vi "Get 1553 Configuration.vi"() -> (3 "1553 Configuration":T1)   [LabVIEW 2020, in "AIM MIL-STD-1553 Engine.lvlib" / "Custom Device.lvlib"]
uses:
  Custom Device.lvlib
  1553 Configuration.ctl
  Major Frame Configuration.ctl
  Minor Frame Configuration.ctl
  Message Configuration.ctl
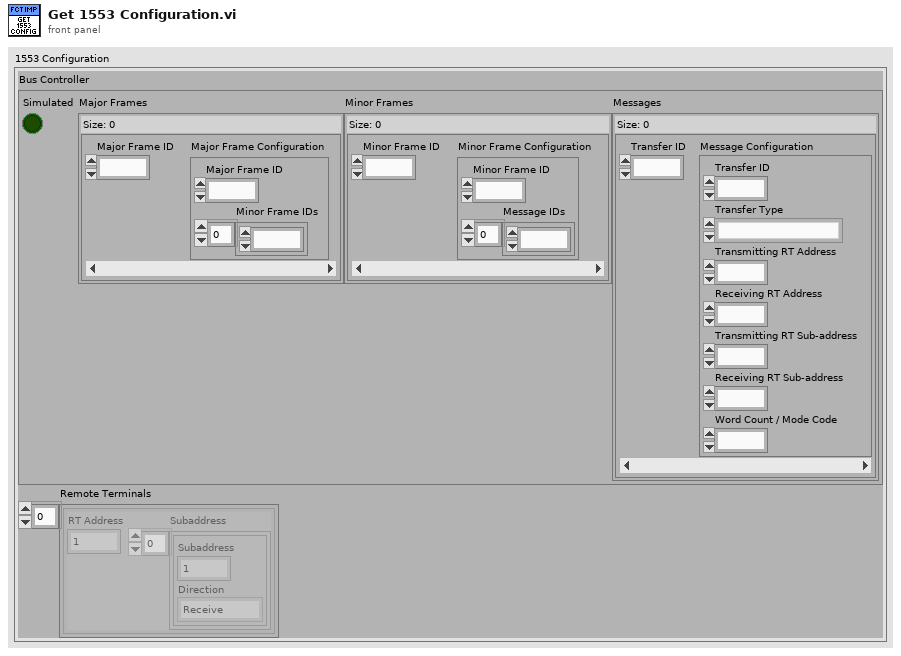
[diagram p1: front panel]
types:
  T1 = typedef "AIM MIL-STD-1553 Engine.lvlib/Custom Device.lvlib/1553 Configuration.ctl" = cluster{"Bus Controller":cluster{"Simulated":bool, "Major Frames":map{u16, T2}, "Minor Frames":map{u16, T3}, "Messages":map{u16, T4}}, "Remote Terminals":cluster{"RT Address":u8, "Subaddress":cluster{"Subaddress":u8, "Direction":enum16{"Receive", "Transmit"}}[]}[]}
  T2 = typedef "AIM MIL-STD-1553 Engine.lvlib/Custom Device.lvlib/Major Frame Configuration.ctl" = cluster{"Major Frame ID":u16, "Minor Frame IDs":u16[]}
  T3 = typedef "AIM MIL-STD-1553 Engine.lvlib/Custom Device.lvlib/Minor Frame Configuration.ctl" = cluster{"Minor Frame ID":u16, "Message IDs":u16[]}
  T4 = typedef "AIM MIL-STD-1553 Engine.lvlib/Custom Device.lvlib/Message Configuration.ctl" = cluster{"Transfer ID":u16, "Transfer Type":enum16{"BC to RT transfer", "RT to BC transfer", "RT to RT transfer"}, "Transmitting RT Address":u8, "Receiving RT Address":u8, "Transmitting RT Sub-address":u8, "Receiving RT Sub-address":u8, "Word Count / Mode Code":u8}
  T5 = cluster{"RT Address":u8, "Subaddress":cluster{"Subaddress":u8, "Direction":enum16{"Receive", "Transmit"}}[]}[]
  T6 = cluster{"Simulated":bool, "Major Frames":map{u16, T2}, "Minor Frames":map{u16, T3}, "Messages":map{u16, T4}}
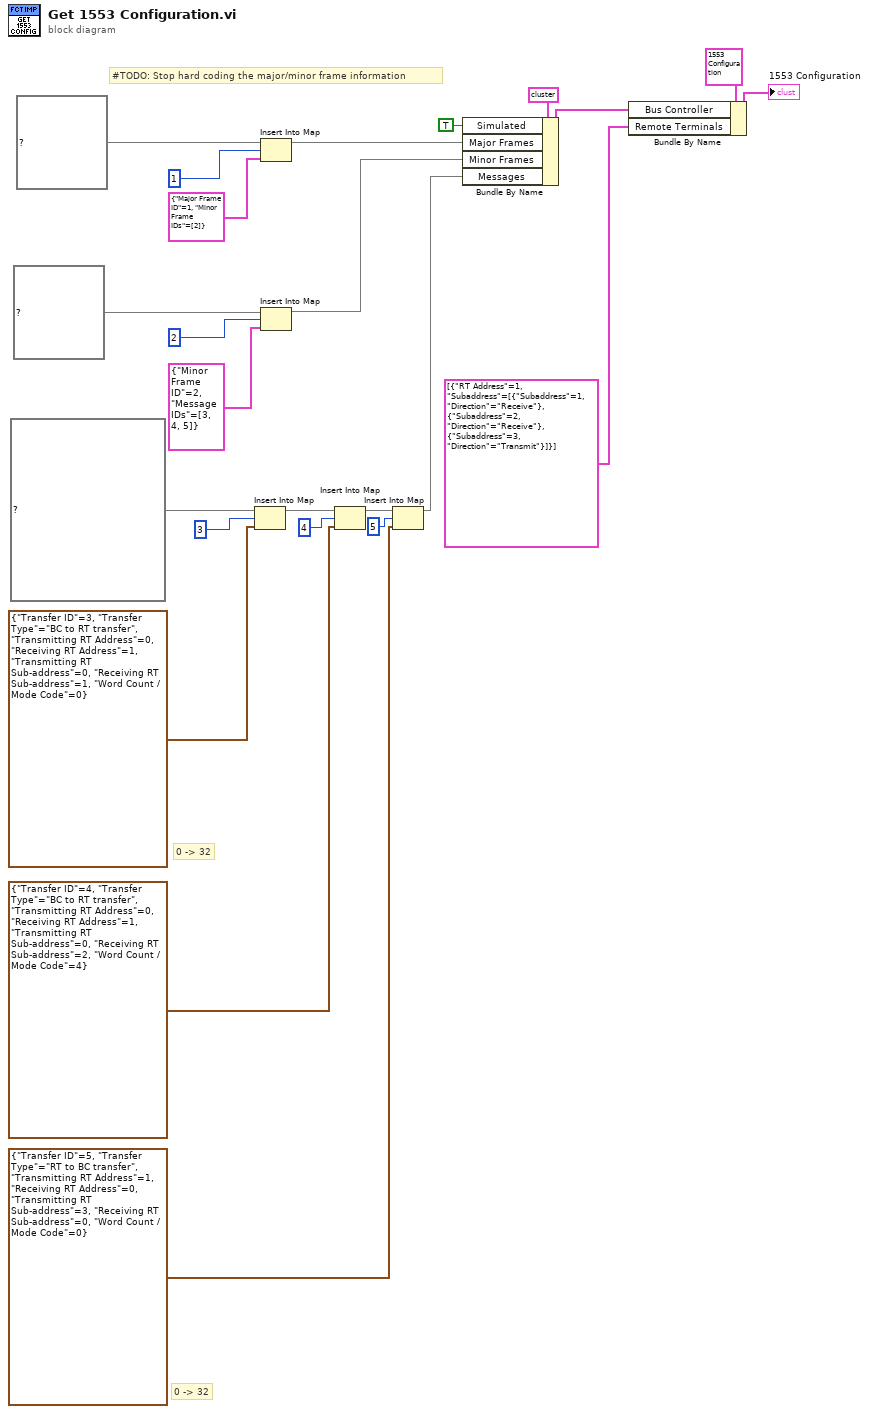
[diagram p0: block diagram]
diagram:
  # "0 -> 32"
  # "#TODO: Stop hard coding the major/minor frame information"
  # "0 -> 32"
  n1 = Insert Into Map(map in=map{u16, T4} {} ("Messages"), key=u16 3, value=T4 {"Transfer ID"=3, "Transfer Type"=enum."BC to RT transfer", "Transmitting RT Address"=0, "Receiving RT Address"=1, "Transmitting RT Sub-address"=0, "Receiving RT Sub-address"=1, "Word Count / Mode Code"=0}) -> (map out=w17:map{u16, T4})  [unwired: 2 out]
  n2 = Insert Into Map(map in=map{u16, T2} {} ("Major Frames"), key=u16 1, value=T2 {"Major Frame ID"=1, "Minor Frame IDs"=[2]}) -> (map out=w6:map{u16, T2})  [unwired: 2 out]
  n3 = Insert Into Map(map in=map{u16, T3} {} ("Minor Frames"), key=u16 2, value=T3 {"Minor Frame ID"=2, "Message IDs"=[3, 4, 5]}) -> (map out=w10:map{u16, T3})  [unwired: 2 out]
  n4 = Insert Into Map(map in=w17, key=u16 4, value=T4 {"Transfer ID"=4, "Transfer Type"=enum."BC to RT transfer", "Transmitting RT Address"=0, "Receiving RT Address"=1, "Transmitting RT Sub-address"=0, "Receiving RT Sub-address"=2, "Word Count / Mode Code"=4}) -> (map out=w20:map{u16, T4})  [unwired: 2 out]
  n5 = Insert Into Map(map in=w20, key=u16 5, value=T4 {"Transfer ID"=5, "Transfer Type"=enum."RT to BC transfer", "Transmitting RT Address"=1, "Receiving RT Address"=0, "Transmitting RT Sub-address"=3, "Receiving RT Sub-address"=0, "Word Count / Mode Code"=0}) -> (map out=w21:map{u16, T4})  [unwired: 2 out]
  n6 = Bundle By Name(cluster=T6 {"Simulated"=FALSE, "Major Frames"={}, "Minor Frames"={}, "Messages"={}} ("Bus Controller"), "Simulated"=TRUE, "Major Frames"=w6, "Minor Frames"=w10, "Messages"=w21) -> (w4:T6)
  n7 = Bundle By Name(cluster=T1 {"Bus Controller"={"Simulated"=FALSE, "Major Frames"={}, "Minor Frames"={}, "Messages"={}}, "Remote Terminals"=[]} ("1553 Configuration"), "Bus Controller"=w4, "Remote Terminals"=T5 [{"RT Address"=1, "Subaddress"=[{"Subaddress"=1, "Direction"=enum."Receive"}, {"Subaddress"=2, "Direction"=enum."Receive"}, {"Subaddress"=3, "Direction"=enum."Transmit"}]}]) -> (→"1553 Configuration":T1)
